vi "HH_ToImageOffline.vi"(0 "Data In":u32[](array[numeric]), 1 "Reset":bool, 2 "Image Array In":i32[][](array[numeric]), 5 "Data Count":i32, 9 "Pixel Time (Laser Pulses)":i32, 11 "Trace Bins":i32=25) -> (3 "Image Array Out":i32[][](array[numeric]), 4 "Histograms":i32[][](array[numeric]), 6 "Total Photon Count":u64[](array[numeric]), 8 "Trigger Times":u64[](array[numeric]), 13 "Total Oveflow Count":u64, 14 "Num Records Total":i64, 15 "Traces":i32[][](array[numeric]))   [LabVIEW 2010]
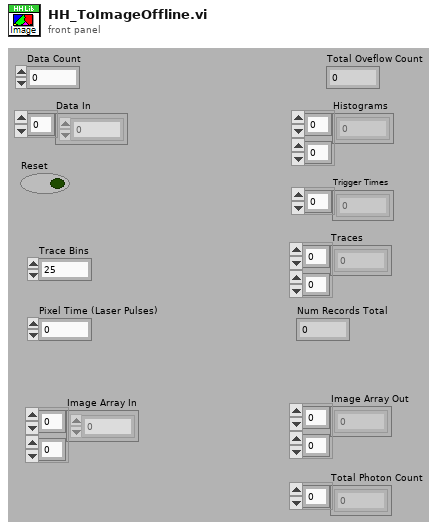
[diagram p1: front panel]
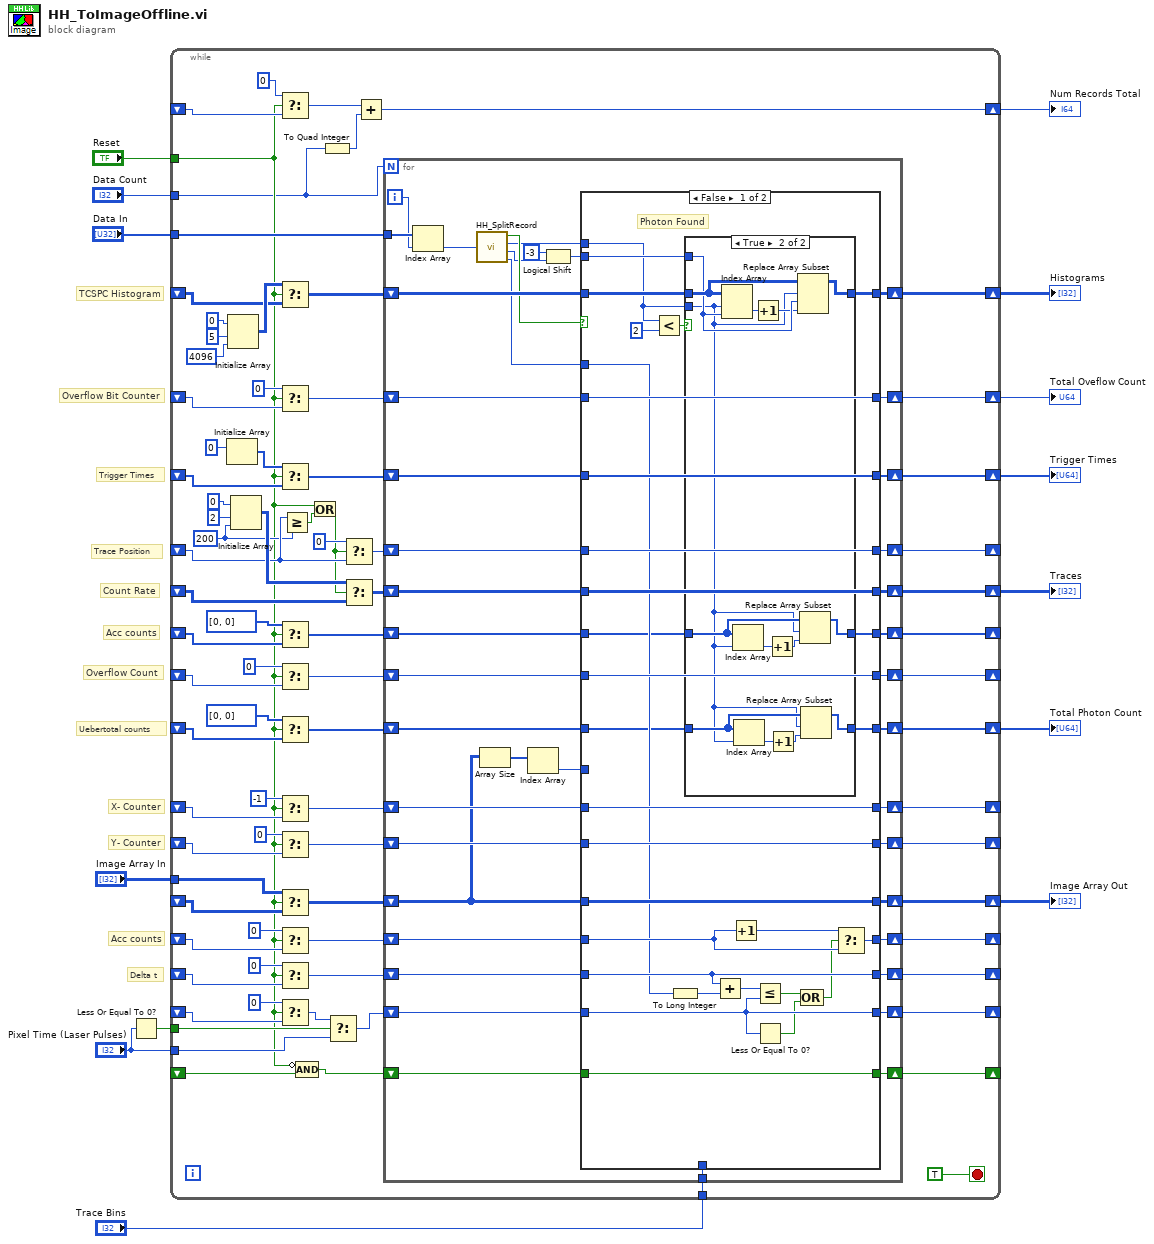
[diagram p0: block diagram]
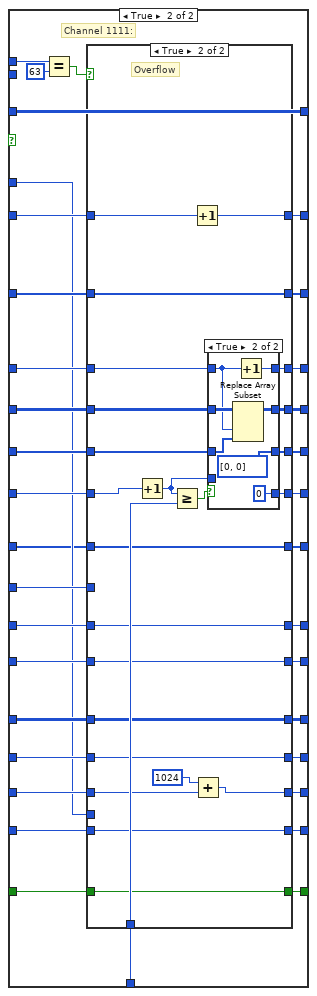
[diagram p3: hidden frame]
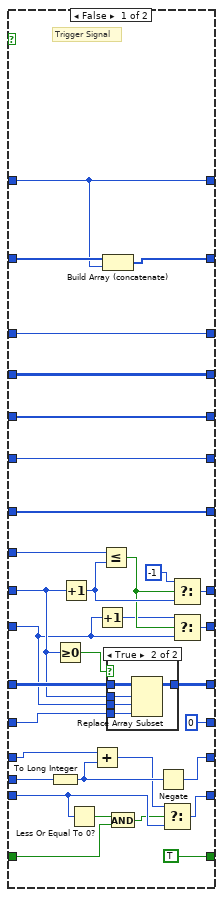
[diagram p4: hidden frame]
diagram:
  # "Uebertotal counts"
  # "Y- Counter"
  # "X- Counter"
  # "Delta t"
  # "Acc counts"
  # "Trace Position"
  # "Overflow Count"
  # "Acc counts"
  # "Count Rate"
  # "Trigger Times"
  # "TCSPC Histogram"
  # "Overflow Bit Counter"
  n1 = Less Or Equal To 0?(x="Pixel Time (Laser Pulses)") -> (x <= 0?=w2:bool)
  n2 = while {
    tunnel: "Data In" -> [w93]
    shift-right: [w94] -> w14
    shift-left: _ -> [w89]
    tunnel: "Reset" -> [w17]
    shift-right: [w86] -> w4
    shift-left: _ -> [w85]
    shift-right: [w81] -> w11
    shift-left: _ -> [w80]
    shift-right: [w76] -> w9
    shift-left: _ -> [w75]
    shift-right: [w73] -> _
    shift-left: _ -> [w72]
    shift-right: [w70] -> _
    shift-left: _ -> [w69]
    tunnel: "Trace Bins" -> [w68]
    shift-right: [w65] -> _
    shift-left: _ -> [w63]
    shift-right: [w59] -> w7
    shift-left: _ -> [w58]
    tunnel: "Image Array In" -> [w61]
    shift-right: [w54] -> _
    shift-left: _ -> [w52]
    shift-right: [w53] -> _
    shift-left: _ -> [w51]
    shift-right: [w46] -> _
    shift-left: _ -> [w44]
    shift-right: [w45] -> _
    shift-left: _ -> [w43]
    tunnel: "Data Count" -> [w16]
    shift-right: [w38] -> w5
    shift-left: _ -> [w40]
    shift-right: [w29] -> w3
    shift-left: _ -> [w28]
    shift-right: [w24] -> _
    shift-left: _ -> [w21]
    tunnel: w2 -> [w26]
    tunnel: "Pixel Time (Laser Pulses)" -> [w25]
    shift-right: [w20] -> _
    shift-left: _ -> [w19]
    stop <- TRUE stop-if-true
    w35 = 200 ("dimension size")
    n3 = Initialize Array(u64 0 ("element")) -> (w83:u64[])  [unwired: 1 out]
    n4 = Initialize Array(0 ("element"), 5 ("dimension size"), 4096 ("dimension size")) -> (w90:i32[][])
    n5 = Initialize Array(0 ("element"), 2 ("dimension size"), w35) -> (w78:i32[][])
    n6 = Select(t=i64 0 ("Data Count 2"), s=w17, f=w40) -> (s? t:f=w39:i64)
    n7 = Select(t=w90, s=w17, f=w89) -> (s? t:f=w91:i32[][])
    n8 = Select(t=u64 0, s=w17, f=w85) -> (s? t:f=w87:u64)
    n9 = Select(t=w83, s=w17, f=w80) -> (s? t:f=w82:u64[])
    n10 = Select(t=u32[] [0, 0] ("initialized array"), s=w17, f=w72) -> (s? t:f=w74:u32[])
    n11 = Select(t=u32 0, s=w17, f=w69) -> (s? t:f=w71:u32)
    n12 = Select(t=u64[] [0, 0] ("initialized array"), s=w17, f=w28) -> (s? t:f=w30:u64[])
    n13 = Select(t=-1, s=w17, f=w44) -> (s? t:f=w48:i32)
    n14 = Select(t=0, s=w17, f=w43) -> (s? t:f=w47:i32)
    n15 = Select(t=w61, s=w17, f=w58) -> (s? t:f=w60:i32[][])
    n16 = Select(t=0, s=w17, f=w52) -> (s? t:f=w56:i32)
    n17 = Select(t=0, s=w17, f=w51) -> (s? t:f=w55:i32)
    n18 = Select(t=0, s=w17, f=w21) -> (s? t:f=w23:i32)
    n19 = Greater Or Equal?(x=w63, y=w35) -> (x >= y?=w64:bool)
    n20 = Compound Arithmetic op=AND(invert w17, w19) -> (w18:bool)
    n21 = Or(x=w17, y=w64) -> (x .or. y?=w62:bool)
    n22 = To Quad Integer(1:w16) -> (0:w15:i64)
    n23 = Select(t=w23, s=w26, f=w25) -> (s? t:f=w27:i32)
    n24 = Select(t=0, s=w62, f=w63) -> (s? t:f=w66:i32)
    n25 = Select(t=w78, s=w62, f=w75) -> (s? t:f=w77:i32[][])
    n26 = Add(x=w39, y=w15) -> (x+y=w38:i64)
    n27 = for {
      N: w16 -> [_]
      tunnel: w93 -> [w109]
      shift-right: [w136] -> w94
      shift-left: w91 -> [w137]
      shift-right: [w134] -> w86
      shift-left: w87 -> [w135]
      shift-right: [w132] -> w81
      shift-left: w82 -> [w133]
      shift-right: [w128] -> w76
      shift-left: w77 -> [w129]
      shift-right: [w130] -> w73
      shift-left: w74 -> [w131]
      shift-right: [w126] -> w70
      shift-left: w71 -> [w127]
      tunnel: w68 -> [w125]
      shift-right: [w123] -> w65
      shift-left: w66 -> [w124]
      shift-right: [w122] -> w59
      shift-left: w60 -> [w114]
      shift-right: [w120] -> w54
      shift-left: w56 -> [w121]
      shift-right: [w118] -> w53
      shift-left: w55 -> [w119]
      shift-right: [w115] -> w46
      shift-left: w48 -> [w116]
      shift-right: [w111] -> w45
      shift-left: w47 -> [w117]
      shift-right: [w106] -> w29
      shift-left: w30 -> [w107]
      shift-right: [w105] -> w24
      shift-left: w27 -> [w110]
      shift-right: [w104] -> w20
      shift-left: w18 -> [w103]
      i -> [w108]
      n28 = Index Array(array=w109, index=w108) -> (element=w102:u32)
      n29 = call "HH_SplitRecord.vi"("Record in"=w102) -> ("Special"=w101:bool, "channel"=w97:i32, "time"=w98:i32, "nsync"=w96:u16)
      n30 = Array Size(array=w114) -> (size(s)=w113:i32[])
      n31 = Index Array(array=w113) -> (element=w112:i32)  [unwired: 1 in]
      n32 = Logical Shift(y=i8 -3, x=w98) -> (x << y=w99:i32)
      n33 = case shown="False" w101 {
        tunnel: w137 -> [w167 w217]
        tunnel: w97 -> [w138 w186]
        tunnel: [w166 w217] -> w136
        tunnel: w99 -> [w139 _]
        tunnel: w135 -> [w165 w219]
        tunnel: [w165 w218] -> w134
        tunnel: w133 -> [w164 w216]
        tunnel: [w164 w215] -> w132
        tunnel: w131 -> [w150 w213]
        tunnel: [w149 w209] -> w130
        tunnel: w129 -> [w163 w212]
        tunnel: [w163 w208] -> w128
        tunnel: w127 -> [w162 w214]
        tunnel: [w162 w210] -> w126
        tunnel: w125 -> [_ w211]
        tunnel: w124 -> [w161 w207]
        tunnel: [w161 w206] -> w123
        tunnel: w114 -> [w160 w204]
        tunnel: [w160 w205] -> w122
        tunnel: w121 -> [w159 w200]
        tunnel: [w158 w201] -> w120
        tunnel: w119 -> [w157 w203]
        tunnel: [w157 w202] -> w118
        tunnel: w117 -> [w156 w199]
        tunnel: w116 -> [w155 w198]
        tunnel: [w155 w197] -> w115
        tunnel: w112 -> [_ w196]
        tunnel: [w156 w195] -> w111
        tunnel: w110 -> [w144 w191]
        tunnel: w96 -> [w152 w194]
        tunnel: w107 -> [w146 w193]
        tunnel: [w145 w192] -> w106
        tunnel: [w144 w190] -> w105
        tunnel: [w140 w189] -> w104
        tunnel: w103 -> [w140 w188]
        frame False {
          # "Photon Found"
          n34 = Less?(x=w138, y=2) -> (x < y?=w148:bool)
          n35 = To Long Integer(number=w152) -> (32bit integer=w151:i32)
          n36 = case shown="True" w148 {
            tunnel: w167 -> [w170 w184]
            tunnel: [w170 w183] -> w166
            tunnel: w139 -> [_ w182]
            tunnel: w138 -> [_ w171]
            tunnel: w150 -> [w169 w181]
            tunnel: [w169 w180] -> w149
            tunnel: w146 -> [w168 w173]
            tunnel: [w168 w172] -> w145
            frame False {
            }
            frame True {
              n37 = Index Array(array=w184, index (row)=w171, index (col)=w182) -> (element=w179:i32)
              n38 = Index Array(array=w181, index=w171) -> (element=w177:u32)
              n39 = Index Array(array=w173, index=w171) -> (element=w175:u64)
              n40 = Increment(x=w179) -> (x+1=w178:i32)
              n41 = Increment(x=w177) -> (x+1=w176:u32)
              n42 = Increment(x=w175) -> (x+1=w174:u64)
              n43 = Replace Array Subset(array=w184, new element=w178, index (row)=w171, index (col)=w182) -> (w183:i32[][])
              n44 = Replace Array Subset(array=w181, new element=w176, index=w171) -> (w180:u32[])
              n45 = Replace Array Subset(array=w173, new element=w174, index=w171) -> (w172:u64[])
            }
          }
          n46 = Add(x=w157, y=w151) -> (x+y=w153:i32)
          n47 = Increment(x=w159) -> (x+1=w154:i32)
          n48 = Less Or Equal?(x=w153, y=w144) -> (x <= y?=w143:bool)
          n49 = Less Or Equal To 0?(x=w144) -> (x <= 0?=w142:bool)
          n50 = Compound Arithmetic op=OR(w143, w142) -> (w141:bool)
          n51 = Select(t=w154, s=w141, f=w159) -> (s? t:f=w158:i32)
        }
        frame True {
          # "Channel 1111:"
          n52 = Equal?(x=w186, y=63) -> (x = y?=w185:bool)
          n53 = case shown="True" w185 {
            tunnel: w219 -> [w250 w281]
            tunnel: [w250 w280] -> w218
            tunnel: w216 -> [w252 w282]
            tunnel: [w251 w282] -> w215
            tunnel: w214 -> [w249 w265]
            tunnel: w213 -> [w248 w276]
            tunnel: w212 -> [w247 w274]
            tunnel: w211 -> [_ w279]
            tunnel: [w249 w277] -> w210
            tunnel: [w248 w275] -> w209
            tunnel: [w247 w273] -> w208
            tunnel: w207 -> [w246 w272]
            tunnel: [w246 w271] -> w206
            tunnel: [w244 w270] -> w205
            tunnel: w204 -> [w245 w270]
            tunnel: w203 -> [w229 w263]
            tunnel: [w231 w259] -> w202
            tunnel: [0 ("t") w268] -> w201
            tunnel: w200 -> [w243 w268]
            tunnel: w194 -> [w228 _]
            tunnel: w199 -> [w233 w267]
            tunnel: w198 -> [w238 w266]
            tunnel: [w240 w266] -> w197
            tunnel: w196 -> [w239 _]
            tunnel: [w234 w267] -> w195
            tunnel: w193 -> [w230 w262]
            tunnel: [w230 w262] -> w192
            tunnel: w191 -> [w225 w261]
            tunnel: [w224 w261] -> w190
            tunnel: [TRUE w260] -> w189
            tunnel: w188 -> [w220 w260]
            frame False {
              # "Trigger Signal"
              n54 = To Long Integer(number=w228) -> (32bit integer=w227:i32)
              n55 = Greater Or Equal To 0?(x=w238) -> (x >= 0?=w241:bool)
              n56 = Increment(x=w238) -> (x+1=w237:i32)
              n57 = Less Or Equal To 0?(x=w225) -> (x <= 0?=w223:bool)
              n58 = Add(x=w229, y=w227) -> (x+y=w226:i32)
              n59 = Increment(x=w233) -> (x+1=w232:i32)
              n60 = Less Or Equal?(x=w239, y=w237) -> (x <= y?=w235:bool)
              n61 = Build Array (concatenate)(w252, w250) -> (w251:u64[])
              n62 = case shown="True" w241 {
                tunnel: w245 -> [w253 w258]
                tunnel: [w253 w257] -> w244
                tunnel: w243 -> [_ w256]
                tunnel: w233 -> [_ w255]
                tunnel: w238 -> [_ w254]
                frame False {
                }
                frame True {
                  n63 = Replace Array Subset(array=w258, new element=w256, index (row)=w254, index (col)=w255) -> (w257:i32[][])
                }
              }
              n64 = And(x=w223, y=w220) -> (x .and. y?=w222:bool)
              n65 = Negate(x=w227) -> (-x=w231:i32)
              n66 = Select(t=w226, s=w222, f=w225) -> (s? t:f=w224:i32)
              n67 = Select(t=-1, s=w235, f=w237) -> (s? t:f=w240:i32)
              n68 = Select(t=w232, s=w235, f=w233) -> (s? t:f=w234:i32)
            }
            frame True {
              # "Overflow"
              n69 = Increment(x=w265) -> (x+1=w264:u32)
              n70 = Greater Or Equal?(x=w264, y=w279) -> (x >= y?=w278:bool)
              n71 = Increment(x=w281) -> (x+1=w280:u64)
              n72 = Add(x=1024 ("t"), y=w263) -> (x+y=w259:i32)
              n73 = case shown="True" w278 {
                tunnel: w264 -> [w286 _]
                tunnel: [w286 u32 0] -> w277
                tunnel: w276 -> [w285 w291]
                tunnel: [w285 u32[] [0, 0] ("initialized array")] -> w275
                tunnel: w274 -> [w284 w292]
                tunnel: [w284 w290] -> w273
                tunnel: w272 -> [w283 w288]
                tunnel: [w283 w289] -> w271
                frame False {
                }
                frame True {
                  n74 = Replace Array Subset(array=w292, new element=w291, index (col)=w288) -> (w290:i32[][])  [unwired: 1 in]
                  n75 = Increment(x=w288) -> (x+1=w289:i32)
                }
              }
            }
          }
        }
      }
    }
  }
  "Histograms" <- w14
  "Trigger Times" <- w11
  "Traces" <- w9
  "Image Array Out" <- w7
  "Num Records Total" <- w5
  "Total Oveflow Count" <- w4
  "Total Photon Count" <- w3
